vi "Prototype.vi"() -> ()   [LabVIEW 2017]
uses:
  <vilib>/FPGAPlugInAG/Dynamic/niLvFpga_Close_Dynamic.vi
  <vilib>/rvi/interface/nirviCloseFPGA/nirviCloseFPGA.xnode
panel:
  out "Error Out":errorcluster
  in  "Bitfile path":path
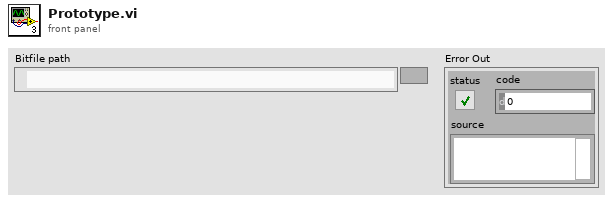
[diagram p1: front panel]
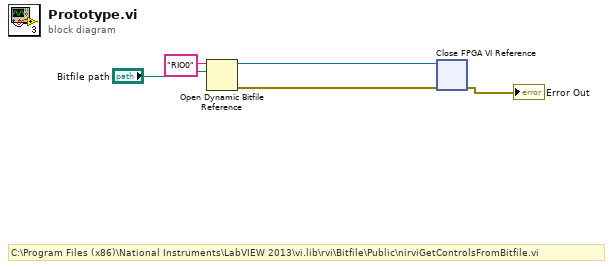
[diagram p0: block diagram]
diagram:
  # "C:\\Program Files (x86)\\National Instruments\\LabVIEW 2013\\vi.lib\\rvi\\Bitfile\\Public\\nirviGetControlsFromBitfile.vi"
  n1 = Open Dynamic Bitfile Reference(0:"RIO0" ("Device address"), 1:"Bitfile path") -> (5:w2:refnum<k20>, 8:w4:errorcluster)  [unwired: 3 in]
  n2 = xnode "Close FPGA VI Reference"("FPGA VI Reference In"=w2, "error in"=w4) -> ("error out"=→"Error Out":errorcluster)
